vi "f_to_c(SubVI).vi"(11 "*F Thermometer":dbl) -> (3 "Numeric":dbl)   [LabVIEW 2015]
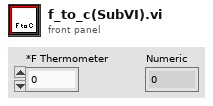
[diagram p1: front panel]
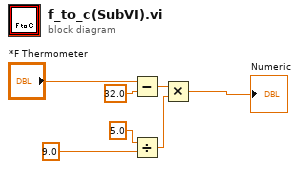
[diagram p0: block diagram]
diagram:
  n1 = Subtract(x="*F Thermometer", y=32.0) -> (x-y=w4:dbl)
  n2 = Divide(x=5.0, y=9.0) -> (x/y=w5:dbl)
  n3 = Multiply(x=w4, y=w5) -> (x*y=→"Numeric":dbl)
